vi "GT Get Watch Var.vi"(7 "pVarInfo":T1, 8 "error in (no error)":errorcluster caption="错误输入（无错误）", 9 "pVar":cluster{"type":u16, "index":u16, "id":u16}, 10 "index":i16, 11 "cardNum":i16) -> (0 "error out":errorcluster caption="错误输出", 1 "pVar out":cluster{"type":u16, "index":u16, "id":u16}, 3 "function return":i16, 5 "pVarInfo out":T1)   [LabVIEW 2020, in "gts1.lvlib"]
doc: "GT_API GT_GetWatchVar(short cardNum,short index,TWatchVar *pVar,TWatchVarInfo *pVarInfo);"
uses:
  gts1.lvlib
  dll/32bit/multi_card/gts.dll
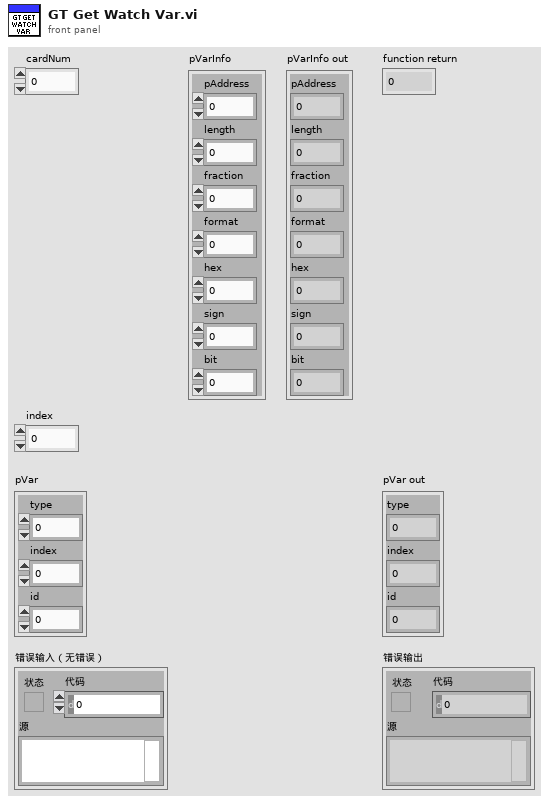
[diagram p1: front panel]
types:
  T1 = cluster{"pAddress":u32, "length":u16, "fraction":i16, "format":u16, "hex":u16, "sign":u16, "bit":u16}
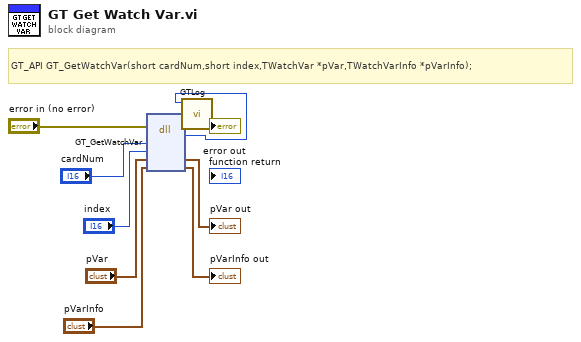
[diagram p0: block diagram]
diagram:
  # "GT_API GT_GetWatchVar(short cardNum,short index,TWatchVar *pVar,TWatchVarInfo *pVarInfo);"
  n1 = dll-call lib="C:/1228/dll/32bit/multi_card/gts.dll" fn="GT_GetWatchVar"(error in="error in (no error)", "cardNum"="cardNum", "index"="index", "pVar"="pVar", "pVarInfo"="pVarInfo") -> (error out=w3:errorcluster, w1:i16, "pVar"=→"pVar out":cluster{"type":u16, "index":u16, "id":u16}, "pVarInfo"=→"pVarInfo out":T1)  [unwired: 4 in, 1 out]
  n2 = call "GTLog.vi"("error in (no error)"=w3, "Numeric"=w1) -> ("error out"=→"error out":errorcluster)  [unwired: 9 in]
